vi "Is Connected.vi"(8 "error in (no error)":errorcluster, 11 "TCP Stream in":refnum<class "TCP Stream.lvclass">) -> (0 "error out":errorcluster, 2 "Connected":bool, 3 "TCP Stream out":refnum<class "TCP Stream.lvclass">)   [LabVIEW 2020, in "Stream-TCP.lvlib" / "TCP Stream.lvclass"]
uses:
  TCP Stream.lvclass
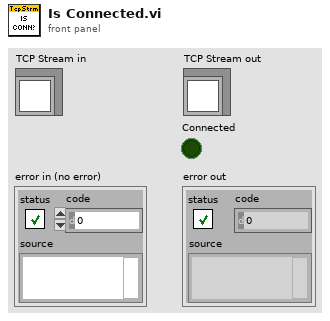
[diagram p1: front panel]
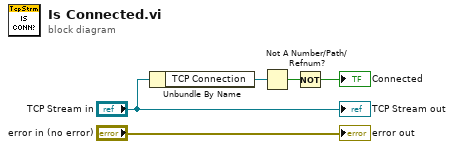
[diagram p0: block diagram]
diagram:
  n1 = Unbundle By Name("TCP Stream in") -> ("TCP Connection"=w3:refnum<k5>)
  n2 = Not A Number/Path/Refnum?(number/path/refnum=w3) -> (NaN/Path/Refnum?=w2:bool)
  n3 = Not(x=w2) -> (.not. x?=→"Connected":bool)
  "error out" <- "error in (no error)"
  "TCP Stream out" <- "TCP Stream in"
